vi "emi_Loop Overview.vi"(0 "Loop index data type":variant, 11 "error in (no error)":errorcluster) -> (8 "Loops":T1[](array[typedef]), 15 "error out":errorcluster)   [LabVIEW 2011]
doc: "gets list of registerd loops.\n\nWire enum to Loop index data type to get loop names"
uses:
  Private/_emi Loop status.ctl
  Private/_emi_Loop control int action.ctl
  <vilib>/Utility/VariantDataType/GetNumericInfo.vi
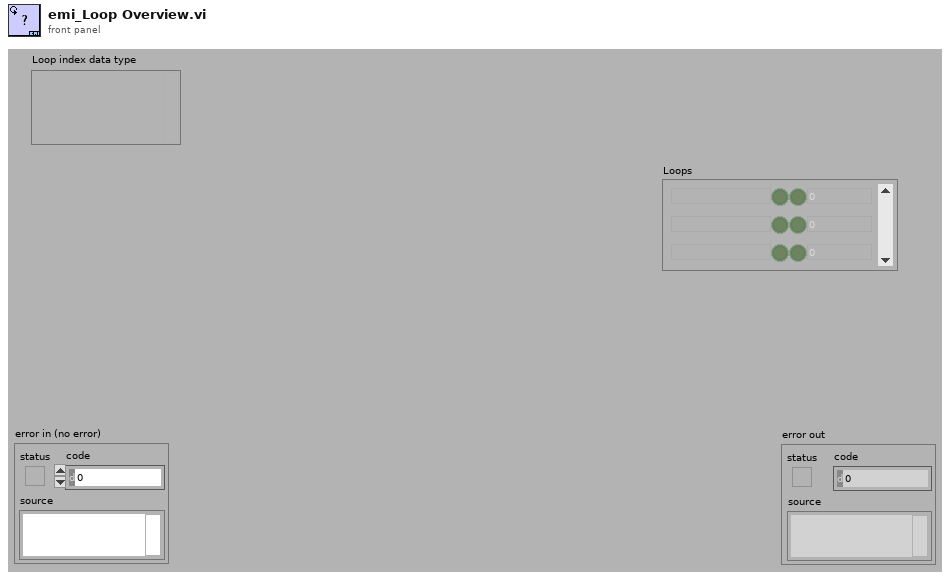
[diagram p1: front panel]
types:
  T1 = typedef "_emi Loop status.ctl" = cluster{"Loop Name":string, "Enabled":bool, "Running":bool, "Restarts":i32}
  T2 = typedef "_emi_Loop control int action.ctl" = enum16{"Init index", "Get index", "Set index", "Get Size"}
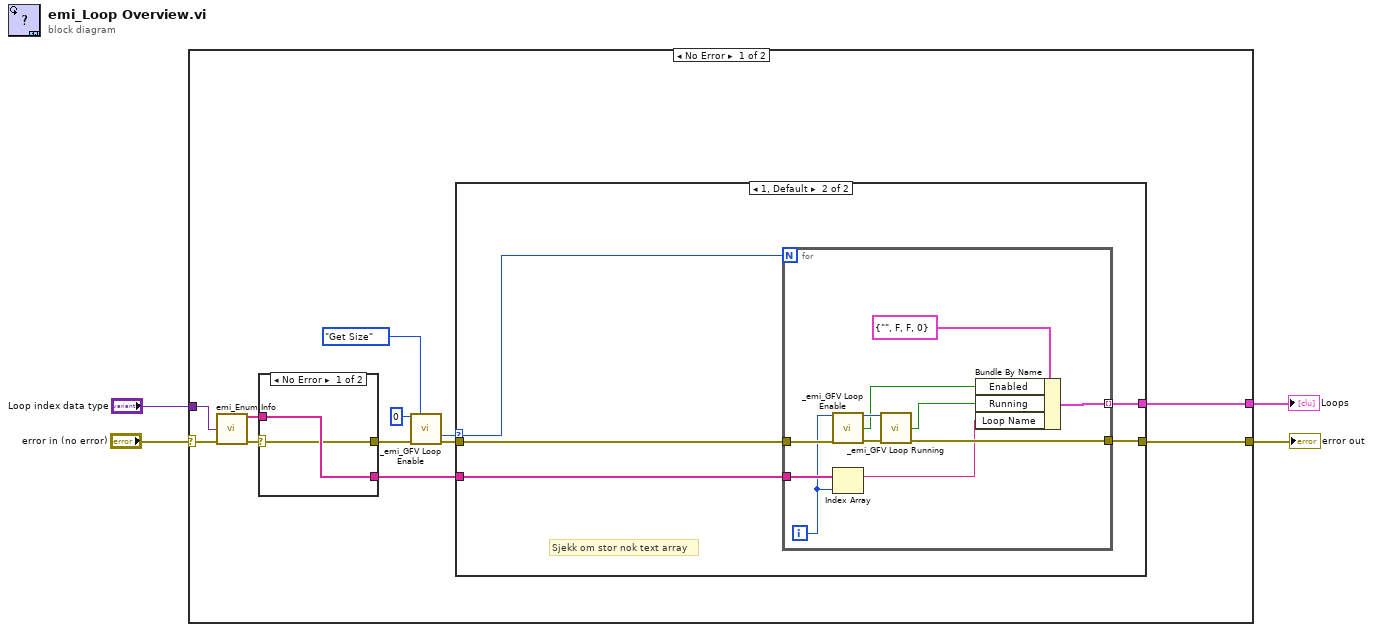
[diagram p0: block diagram]
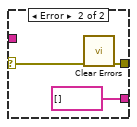
[diagram p2: hidden frame]
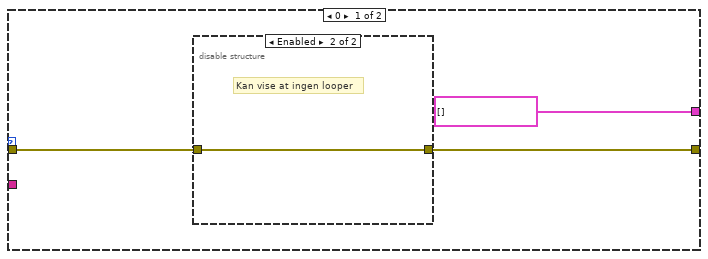
[diagram p3: hidden frame]
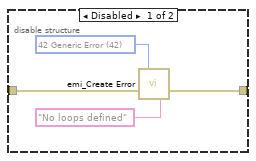
[diagram p4: hidden frame]
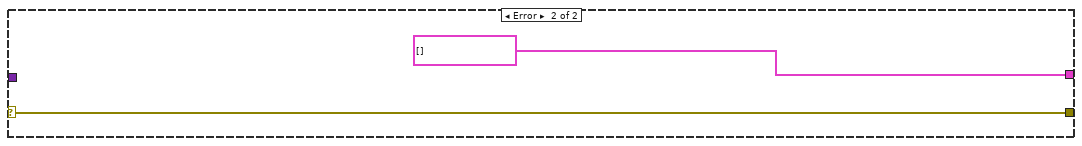
[diagram p5: hidden frame]
diagram:
  n1 = case shown="No Error" "error in (no error)" {
    selector: "error in (no error)" -> [w9 w47]
    tunnel: [w12 w47] -> w3
    tunnel: "Loop index data type" -> [w11 _]
    tunnel: [w5 T1[] []] -> w1
    frame No Error {
      n2 = call "emi_Enum Info.vi"("Enum"=w11, "error in (no error)"=w9) -> ("Text Elements"=w7:string[], "error out"=w10:errorcluster)  [unwired: 10 in, 2 out]
      n3 = case shown="No Error" w10 {
        selector: w10 -> [w17 w21]
        tunnel: [w17 w20] -> w8
        tunnel: w7 -> [w18 _]
        tunnel: [w18 string[] [] ("Text Elements")] -> w6
        frame No Error {
        }
        frame Error {
          n4 = call <vilib>:"Clear Errors.vi"("error in (no error)"=w21) -> ("error out"=w20:errorcluster)  [unwired: 6 in]
        }
      }
      n5 = call "_emi_GFV Loop Enable.vi"("Loop Index/Numb"=u16 0 ("Dummy"), "Action(Get Index)"=_emi_Loop_control_int_action."Get Size", "error in (no error)"=w8) -> ("Size"=w15:i32, "error out"=w14:errorcluster)  [unwired: 9 in, 2 out]
      n6 = case shown="1, Default" w15 {
        selector: w15 -> [_ w34]
        tunnel: w14 -> [w24 w33]
        tunnel: [w23 w31] -> w12
        tunnel: w6 -> [_ w32]
        tunnel: [T1[] [] w30] -> w5
        frame 0 {
          n7 = disable-structure shown="Enabled" {
            disable-tunnel: w24 -> [w26 w29]
            disable-tunnel: [w25 w29] -> w23
            frame Disabled {
              w28 = 42 items=["0 No Error"=0, "1 Invalid input parameter"=1, "6 Generic file IO "=6, "7 File not Found"=7, "35 Generic Pring Error"=35, "37 Device not Found"=37, "39 Device Unit Error"=39, "40 Could fot Open Device"=40, "42 Generic Error"=42, "52 Unknown Message"=52, "98 Bad File type"=98, "99 Bad File Version"=99, "100 Bad Data in File"=100, "1018 Unspecefied Error"=1018, "1041 Incorrect Password"=1041, "1043 Feature not in this version"=1043, "1109 Unsuported Data type"=1109, "1444 Did not close sucessfully"=1444] ("Error Code")
              n8 = call "emi_Create Error.vi"("Error Code"=w28, "error in (no error)"=w26, "Append String(\"\")"="No loops defined" ("Append String(\"\")")) -> ("error out"=w25:errorcluster)  [unwired: 12 in]
            }
            frame Enabled {
              # "Kan vise at ingen looper"
            }
          }
        }
        frame 1, Default {
          # "Sjekk om stor nok text array"
          n9 = for {
            N: w34 -> [_]
            tunnel: w33 -> [w45]
            tunnel: w32 -> [w39]
            tunnel: [w38] -> w31
            tunnel: [w37] -> w30 mode=indexing
            i -> [w35]
            n10 = call "_emi_GFV Loop Enable.vi"("Loop Index/Numb"=w35, "error in (no error)"=w45) -> ("Index out"=w43:u16, "Loop Enable Out"=w41:bool, "error out"=w44:errorcluster)  [unwired: 10 in, 1 out]
            n11 = Index Array(array=w39, index=w35) -> (element=w36:string)
            n12 = call "_emi_GFV Loop Running.vi"("Loop Index/Numb"=w43, "error in (no error)"=w44) -> ("Loop Running Out"=w40:bool, "error out"=w38:errorcluster)  [unwired: 10 in, 2 out]
            n13 = Bundle By Name(cluster=T1 {"Loop Name"="", "Enabled"=FALSE, "Running"=FALSE, "Restarts"=0} ("Loop status"), "Enabled"=w41, "Running"=w40, "Loop Name"=w36) -> (w37:T1)
          }
        }
      }
    }
    frame Error {
    }
  }
  "error out" <- w3
  "Loops" <- w1
